vi "SPD.Update SPD Type.vi"(4 "Gate SPD ctrls":refnum<vi>[](array[refnum]), 6 "General SPD ctrls":refnum<vi>[](array[refnum]), 7 "SPD config base name":string="SPDConfig", 8 "error in (no error)":errorcluster, 10 "specification":T1, 11 "SPD.Stand Ctrl in":T5 {"spdDeviceSession"."hidSPD.Sturtup Values"."HV_bias" format="%#_6p, V"; "spdDeviceSession"."hidSPD.Sturtup Values"."TSet" format="%#_6p, DegC"; "spdDeviceSession"."hidSPD.Controller"."HV_bias" format="%#_6p, V"; "spdDeviceSession"."hidSPD.Controller"."TSet" format="%#_6p, DegC"}) -> (0 "error out":errorcluster, 3 "SPD.Stand Ctrl out":T5 {"spdDeviceSession"."hidSPD.Sturtup Values"."HV_bias" format="%#_6p, V"; "spdDeviceSession"."hidSPD.Sturtup Values"."TSet" format="%#_6p, DegC"; "spdDeviceSession"."hidSPD.Controller"."HV_bias" format="%#_6p, V"; "spdDeviceSession"."hidSPD.Controller"."TSet" format="%#_6p, DegC"})   [LabVIEW 2018]
uses:
  typedefs/SPD.Stand Ctrl.ctl
  Instruments/SPD HID Interface/hidSPDLibForLabView/LibVIs/hidSPD Controls/hidSPD Device Session.ctl
  Instruments/SPD HID Interface/hidSPDLibForLabView/LibVIs/hidSPD Controls/hidSPD.SPD specification.ctl
  Instruments/SPD HID Interface/hidSPDLibForLabView/LibVIs/hidSPD Controls/hidSPD SPD Diod Case.ctl
  Instruments/SPD HID Interface/hidSPDLibForLabView/LibVIs/hidSPD Controls/hidSPD SPD Type.ctl
  Instruments/SPD HID Interface/hidSPDLibForLabView/LibVIs/hidSPD Controls/hidSPD.STB Frequency.ctl
  Instruments/SPD HID Interface/hidSPDLibForLabView/LibVIs/hidSPD Controls/hidSPD Controller.ctl
  Instruments/KC705 DevBoard/typedefs/DevB.Session.ctl
  Instruments/KeySight 53230A/typedefs/FreqC.Session.ctl
  Instruments/KeySight 8164B/KeySight 8164B LAN InstrLib/typedefs/KeySight 8164B control.ctl
  Instruments/LeCroy SDA830/typedefs/LeCroy.Session.ctl
  typedefs/SPD.Events.ctl
  ConfigFile/SPD.Config File ctrl.ctl
  <vilib>/Utility/config.llb/Config Data RefNum.ctl
  typedefs/SPD.Meas Grid.ctl
  typedefs/SPD.Queues.ctl
  typedefs/SPD.Stand state.ctl
  Instruments/KeySight 8164B/KeySight 8164B LAN InstrLib.lvlib
  <vilib>/Utility/config.llb/NI_LVConfig.lvlib
  Instruments/SPD HID Interface/hidSPDLibForLabView/hidSPDLibForLabView.lvlib
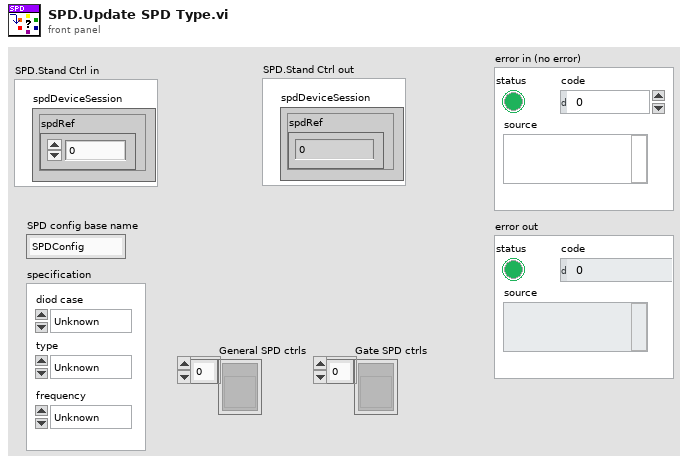
[diagram p1: front panel]
types:
  T1 = typedef "hidSPDLibForLabView.lvlib/hidSPD.SPD specification.ctl" = cluster{"diod case":T2, "type":T3, "frequency":T4}
  T2 = typedef "hidSPDLibForLabView.lvlib/hidSPD SPD Diod Case.ctl" = enum16{"Unknown", "default", "butterfly"}
  T3 = typedef "hidSPDLibForLabView.lvlib/hidSPD SPD Type.ctl" = enum16{"Unknown", "Free Run", "Gate"}
  T4 = typedef "hidSPDLibForLabView.lvlib/hidSPD.STB Frequency.ctl" = enum16{"Unknown", "312", "1250"}
  T5 = typedef "SPD.Stand Ctrl.ctl" = cluster{"spdDeviceSession":T6, "DevBSession":T8, "FreqCSession":T9, "8164BSession":T10, "LeCroySession":T11, "Events":T12, "configFile":T13, "SPD.Meas Grid":T15, "SPD.Queues":T16, "Console":refnum<vi>}
  T6 = typedef "hidSPDLibForLabView.lvlib/hidSPD Device Session.ctl" = cluster{"spdRef":u64, "connected":bool, "spdName":string, "specification":T1, "hidSPD.Controller":T7, "hidSPD.Sturtup Values":T7}
  T7 = typedef "hidSPDLibForLabView.lvlib/hidSPD Controller.ctl" = cluster{"TSet":sgl, "HV_bias":sgl, "DDS_stb_code":u16}
  T8 = typedef "DevB.Session.ctl" = cluster{"DevBRef":refnum<visa-resource-name>, "connected":bool}
  T9 = typedef "FreqC.Session.ctl" = cluster{"FreqCRef":refnum<visa-resource-name>, "timeout":dbl, "Gate":dbl, "connected":bool}
  T10 = typedef "KeySight 8164B LAN InstrLib.lvlib/KeySight 8164B control.ctl" = cluster{"Connection ID":refnum<k5>, "Connected":bool, "Info":string, "Slots Info":string[]}
  T11 = typedef "LeCroy.Session.ctl" = cluster{"LeCroySession":refnum<visa-resource-name>, "connected":bool}
  T12 = typedef "SPD.Events.ctl" = cluster{"DCRTest":refnum<user-event>, "Stop":refnum<user-event>}
  T13 = typedef "SPD.Config File ctrl.ctl" = cluster{"configFile ref":T14, "configFile path":path, "equipmentFile ref":T14}
  T14 = typedef "NI_LVConfig.lvlib/Config Data RefNum.ctl" = refnum<k1>
  T15 = typedef "SPD.Meas Grid.ctl" = cluster{"DateTime":string, "DT":dbl[], "Insensitivity":dbl[], "Temprature":dbl[], "Stb_code":dbl[], "HV_Bias":dbl[][][][]}
  T16 = typedef "SPD.Queues.ctl" = cluster{"state queue":refnum<queue>}
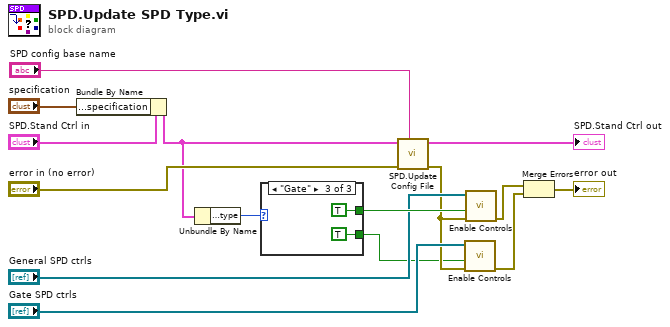
[diagram p0: block diagram]
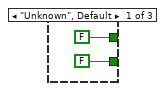
[diagram p2: hidden frame]
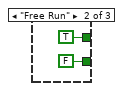
[diagram p3: hidden frame]
diagram:
  n1 = Bundle By Name(cluster="SPD.Stand Ctrl in", "spdDeviceSession.specification"="specification") -> (w2:T5)
  n2 = Unbundle By Name(w2) -> ("spdDeviceSession.specification.type"=w1:T3)
  n3 = case shown="\"Gate\"" w1 {
    tunnel: [FALSE FALSE TRUE] -> w8
    tunnel: [FALSE TRUE TRUE] -> w15
    frame "Unknown", Default {
    }
    frame "Free Run" {
    }
    frame "Gate" {
    }
  }
  n4 = call "SPD.Update Config File.vi"("SPD config base name"="SPD config base name", "Error In"="error in (no error)", "SPD.Stand Ctrl in"=w2) -> ("Error Out"=w9:errorcluster, "SPD.Stand Ctrl out"=→"SPD.Stand Ctrl out":T5)  [unwired: 7 in]
  n5 = call "Enable Controls.vi"("error in (no error)"=w9, "enable"=w8, "Control"="Gate SPD ctrls") -> ("error out"=w10:errorcluster)  [unwired: 8 in]
  n6 = call "Enable Controls.vi"("error in (no error)"=w9, "enable"=w15, "Control"="General SPD ctrls") -> ("error out"=w12:errorcluster)  [unwired: 8 in]
  n7 = Merge Errors(w12, w10) -> (→"error out":errorcluster)
